vi "Read UI Constants.vi"(8 "error in":errorcluster, 11 "CFG File Refnum in":T2) -> (0 "error out":errorcluster, 2 "MHL Configuration":T1, 3 "CFG File Refnum out":T2)   [LabVIEW 2020]
uses:
  <vilib>/Utility/config.llb/Config Data RefNum.ctl
  controls/MHL Configuration.ctl
  Boiler System Globals.vi
  <vilib>/Utility/config.llb/Read Key (Double).vi
  <vilib>/Utility/error.llb/Error Cluster From Error Code.vi
  <vilib>/ErrorRing/Error Ring.xnode
  <vilib>/Utility/config.llb/NI_LVConfig.lvlib
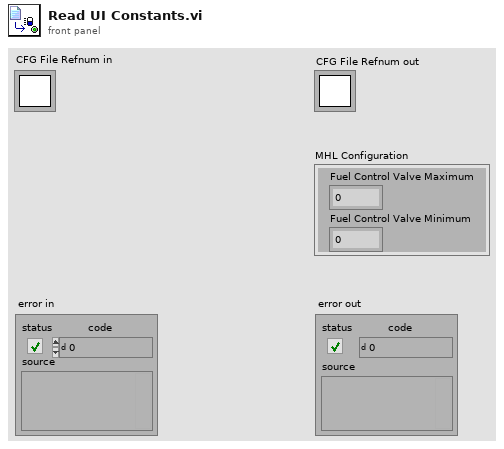
[diagram p1: front panel]
types:
  T1 = typedef "MHL Configuration.ctl" = cluster{"Fuel Control Valve Maximum":dbl, "Fuel Control Valve Minimum":dbl}
  T2 = typedef "NI_LVConfig.lvlib/Config Data RefNum.ctl" = refnum<k1>
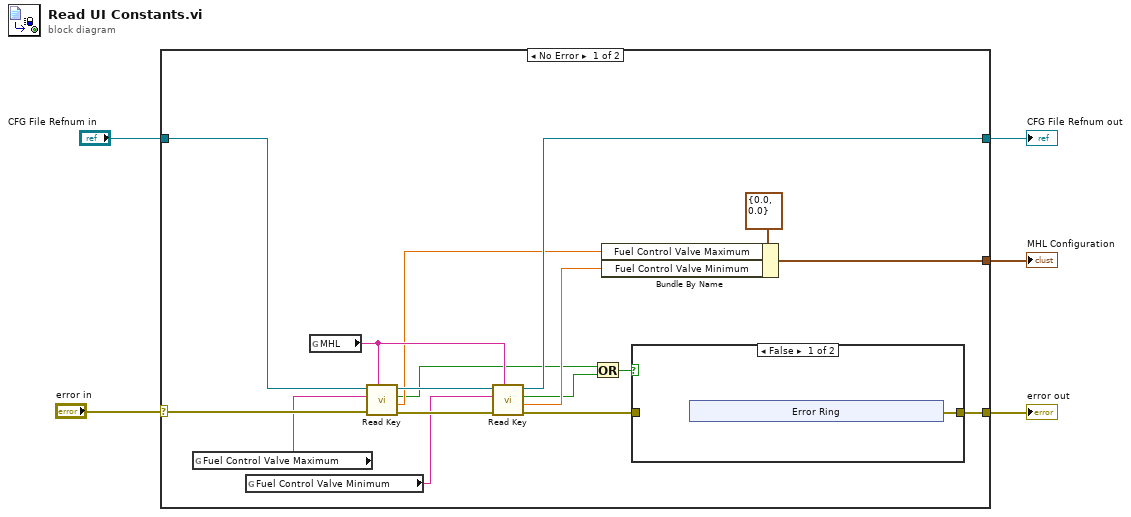
[diagram p0: block diagram]
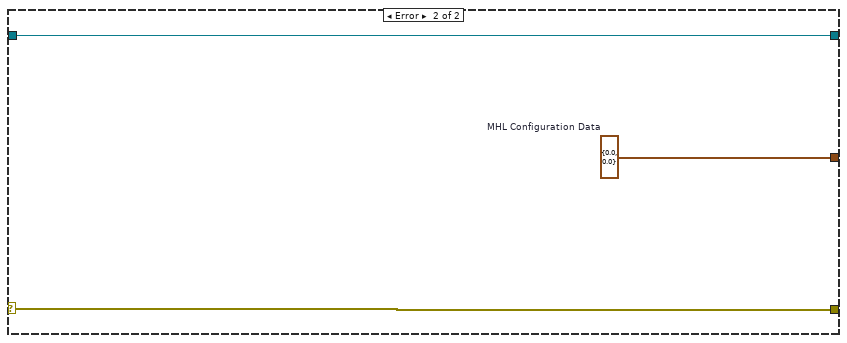
[diagram p3: hidden frame]
diagram:
  n1 = case shown="No Error" "error in" {
    selector: "error in" -> [w22 w32]
    tunnel: [w9 w32] -> w4
    tunnel: "CFG File Refnum in" -> [w19 w31]
    tunnel: [w17 w31] -> w2
    tunnel: [w11 w30] -> w1
    frame No Error {
      n2 = global read "Boiler System Globals.vi" "Fuel Control Valve Maximum"() -> (w16:string)
      n3 = global read "Boiler System Globals.vi" "Fuel Control Valve Minimum"() -> (w15:string)
      n4 = global read "Boiler System Globals.vi" "MHL"() -> (w20:string)
      n5 = call-poly <vilib>:"Read Key.vi"("section"=w20, "error in (no error)"=w22, "key"=w16, "refnum"=w19) -> ("error out"=w21:errorcluster, "value"=w13:dbl, "found?"=w8:bool, "refnum out"=w18:T2)  [unwired: 4 in]
      n6 = call-poly <vilib>:"Read Key.vi"("section"=w20, "error in (no error)"=w21, "key"=w15, "refnum"=w18) -> ("error out"=w10:errorcluster, "value"=w12:dbl, "found?"=w7:bool, "refnum out"=w17:T2)  [unwired: 4 in]
      n7 = Or(x=w8, y=w7) -> (x .or. y?=w6:bool)
      n8 = Bundle By Name(cluster=T1 {"Fuel Control Valve Maximum"=0.0, "Fuel Control Valve Minimum"=0.0} ("MHL Configuration"), "Fuel Control Valve Maximum"=w13, "Fuel Control Valve Minimum"=w12) -> (w11:T1)
      n9 = case shown="False" w6 {
        tunnel: w10 -> [_ w29]
        tunnel: [w23 w29] -> w9
        frame False {
          n10 = xnode "Error Ring"() -> ("error out"=w23:errorcluster)
        }
        frame True {
        }
      }
    }
    frame Error {
      w30 = T1 {"Fuel Control Valve Maximum"=0.0, "Fuel Control Valve Minimum"=0.0}  # MHL Configuration Data
    }
  }
  "error out" <- w4
  "CFG File Refnum out" <- w2
  "MHL Configuration" <- w1
